vi "Insts_post.vi"(2 "Initialize sweep instruments ??":u64[](array[numeric]), 4 "Initialize readout instruments??":u64[](array[numeric]), 5 "Inst_array":T1(array[cluster])) -> ()   [LabVIEW 2013]
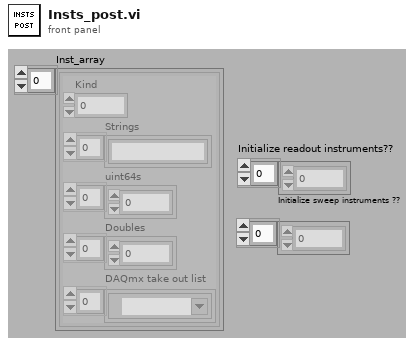
[diagram p1: front panel]
types:
  T1 = cluster{"Kind":u16, "Strings":string[], "uint64s":u64[], "Doubles":dbl[], "DAQmx take out list":refnum<k21>[]}[]
  T2 = cluster{"Kind":u16, "Strings":string[], "uint64s":u64[], "Doubles":dbl[], "DAQmx take out list":refnum<k21>[]}
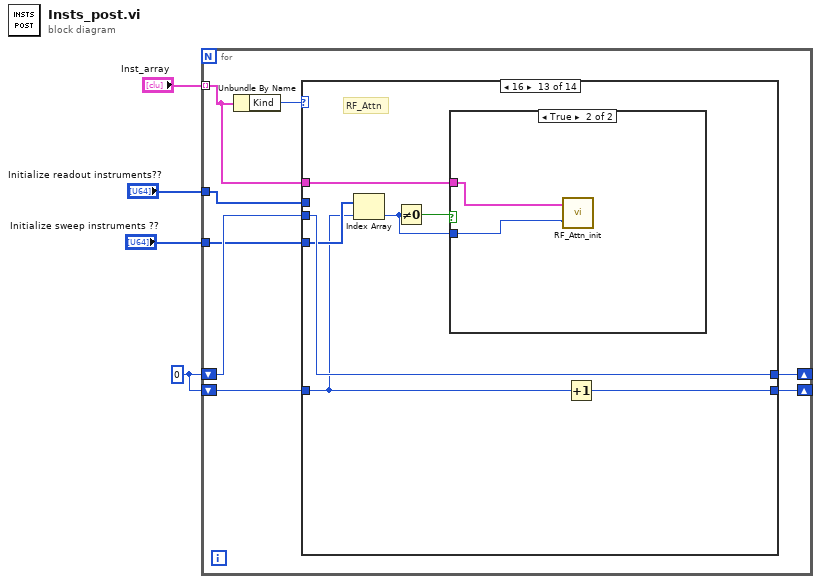
[diagram p0: block diagram]
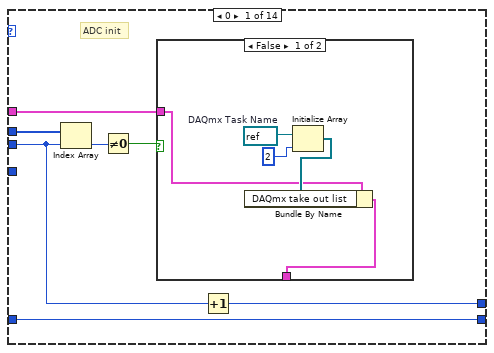
[diagram p2: hidden frame]
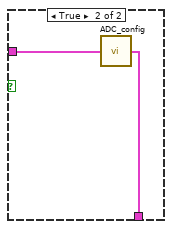
[diagram p3: hidden frame]
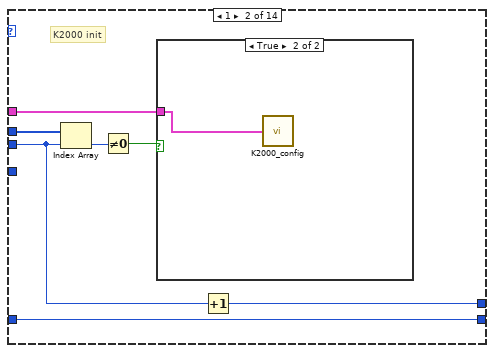
[diagram p4: hidden frame]
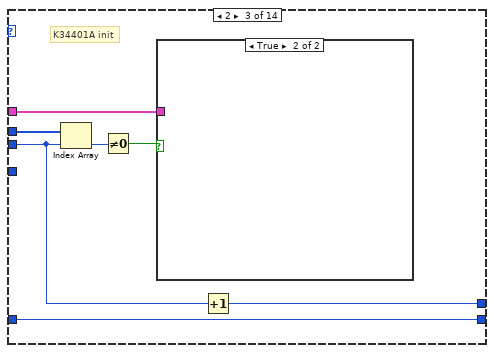
[diagram p6: hidden frame]
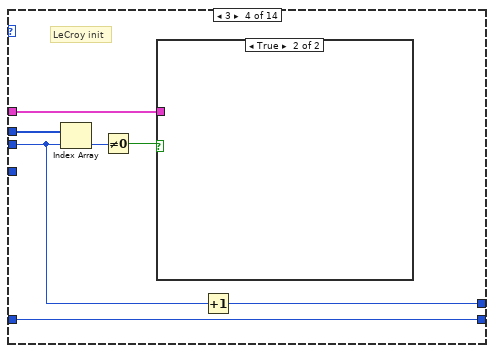
[diagram p8: hidden frame]
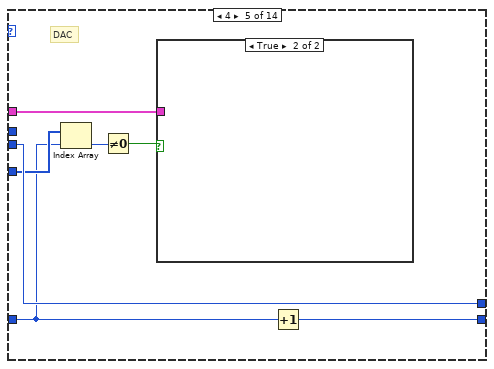
[diagram p10: hidden frame]
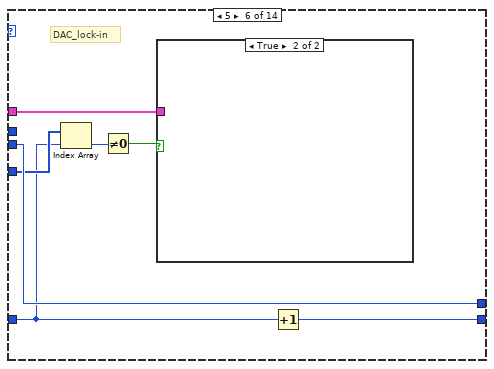
[diagram p12: hidden frame]
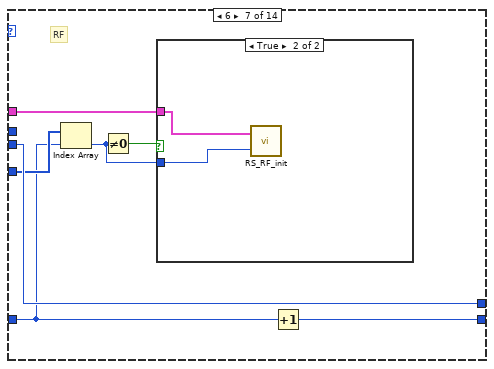
[diagram p14: hidden frame]
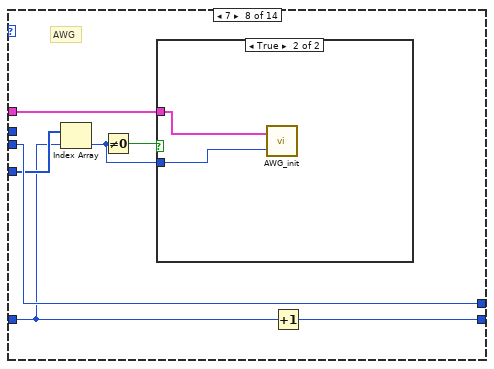
[diagram p16: hidden frame]
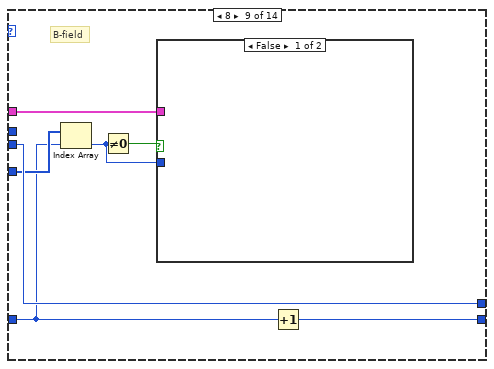
[diagram p18: hidden frame]
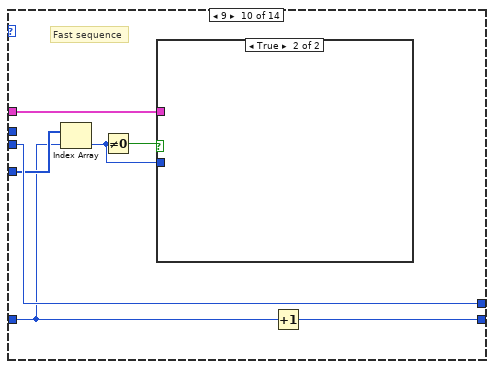
[diagram p20: hidden frame]
diagram:
  w1 = 0
  n1 = for {
    tunnel: "Inst_array" -> [w9] mode=indexing
    tunnel: "Initialize sweep instruments ??" -> [w6]
    tunnel: "Initialize readout instruments??" -> [w10]
    shift-right: [w8] -> _
    shift-left: w1 -> [w11]
    shift-right: [w5] -> _
    shift-left: w1 -> [w7]
    n2 = Unbundle By Name(w9) -> ("Kind"=w12:u16)
    n3 = case shown="16" w12 {
      tunnel: w11 -> [w15 w30 w38 w45 w53 w60 w68 w77 w86 w93 w100 w107 w114 w119]
      tunnel: w10 -> [w19 w33 w41 w48 _ _ _ _ _ _ _ _ _ _]
      tunnel: w9 -> [w16 w28 w36 w43 w49 w56 w64 w73 w82 w89 w96 w103 w110 _]
      tunnel: [w14 w29 w37 w44 w53 w60 w68 w77 w86 w93 w100 w107 w114 w119] -> w8
      tunnel: w7 -> [w13 w27 w35 w42 w50 w57 w65 w74 w83 w90 w97 w104 w111 w118]
      tunnel: w6 -> [_ _ _ _ w52 w59 w67 w76 w85 w92 w99 w106 w113 _]
      tunnel: [w13 w27 w35 w42 w51 w58 w66 w75 w84 w91 w98 w105 w112 w118] -> w5
      frame 0 {
        # "ADC init"
        n4 = Index Array(array=w19, index=w15) -> (element=w18:u64)
        n5 = Not Equal To 0?(x=w18) -> (x != 0?=w17:bool)
        n6 = case shown="False" w17 {
          tunnel: w16 -> [w21 w26]
          tunnel: [w20 w25] -> _
          frame False {
            w24 = refnum<k21> refnum  # DAQmx Task Name
            n7 = Initialize Array(w24, 2) -> (w22:refnum<k21>[])
            n8 = Bundle By Name(cluster=w21, "DAQmx take out list"=w22) -> (w20:T2)
          }
          frame True {
            n9 = call "ADC_config.vi"("Inst_parameter"=w26) -> ("Inst_parameter out"=w25:T2)
          }
        }
        n10 = Increment(x=w15) -> (x+1=w14:i32)
      }
      frame 1 {
        # "K2000 init"
        n11 = Index Array(array=w33, index=w30) -> (element=w32:u64)
        n12 = Not Equal To 0?(x=w32) -> (x != 0?=w31:bool)
        n13 = case shown="True" w31 {
          tunnel: w28 -> [_ w34]
          frame False {
          }
          frame True {
            n14 = call "K2000_config.vi"("Readout_inst_parameters"=w34) -> ()  [unwired: 1 out]
          }
        }
        n15 = Increment(x=w30) -> (x+1=w29:i32)
      }
      frame 2 {
        # "K34401A init"
        n16 = Index Array(array=w41, index=w38) -> (element=w40:u64)
        n17 = Not Equal To 0?(x=w40) -> (x != 0?=w39:bool)
        n18 = case shown="True" w39 {
          tunnel: w36 -> [_ _]
          frame False {
          }
          frame True {
          }
        }
        n19 = Increment(x=w38) -> (x+1=w37:i32)
      }
      frame 3 {
        # "LeCroy init"
        n20 = Index Array(array=w48, index=w45) -> (element=w47:u64)
        n21 = Not Equal To 0?(x=w47) -> (x != 0?=w46:bool)
        n22 = case shown="True" w46 {
          tunnel: w43 -> [_ _]
          frame False {
          }
          frame True {
          }
        }
        n23 = Increment(x=w45) -> (x+1=w44:i32)
      }
      frame 4 {
        # "DAC"
        n24 = Index Array(array=w52, index=w50) -> (element=w55:u64)
        n25 = Not Equal To 0?(x=w55) -> (x != 0?=w54:bool)
        n26 = case shown="True" w54 {
          tunnel: w49 -> [_ _]
          frame False {
          }
          frame True {
          }
        }
        n27 = Increment(x=w50) -> (x+1=w51:i32)
      }
      frame 5 {
        # "DAC_lock-in"
        n28 = Index Array(array=w59, index=w57) -> (element=w62:u64)
        n29 = Not Equal To 0?(x=w62) -> (x != 0?=w61:bool)
        n30 = case shown="True" w61 {
          tunnel: w56 -> [_ _]
          frame False {
          }
          frame True {
          }
        }
        n31 = Increment(x=w57) -> (x+1=w58:i32)
      }
      frame 6 {
        # "RF"
        n32 = Index Array(array=w67, index=w65) -> (element=w63:u64)
        n33 = Not Equal To 0?(x=w63) -> (x != 0?=w69:bool)
        n34 = case shown="True" w69 {
          tunnel: w64 -> [_ w71]
          tunnel: w63 -> [_ w70]
          frame False {
          }
          frame True {
            n35 = call "RS_RF_init.vi"("Initialize Instrument"=w70, "Inst_param"=w71) -> ()  [unwired: 1 in]
          }
        }
        n36 = Increment(x=w65) -> (x+1=w66:i32)
      }
      frame 7 {
        # "AWG"
        n37 = Index Array(array=w76, index=w74) -> (element=w72:u64)
        n38 = Not Equal To 0?(x=w72) -> (x != 0?=w78:bool)
        n39 = case shown="True" w78 {
          tunnel: w73 -> [_ w80]
          tunnel: w72 -> [_ w79]
          frame False {
          }
          frame True {
            n40 = call "AWG_init.vi"("Initialize?"=w79, "Inst_param"=w80) -> ()  [unwired: 1 out]
          }
        }
        n41 = Increment(x=w74) -> (x+1=w75:i32)
      }
      frame 8 {
        # "B-field"
        n42 = Index Array(array=w85, index=w83) -> (element=w81:u64)
        n43 = Not Equal To 0?(x=w81) -> (x != 0?=w87:bool)
        n44 = case shown="False" w87 {
          tunnel: w82 -> [_ _]
          tunnel: w81 -> [_ _]
          frame False {
          }
          frame True {
          }
        }
        n45 = Increment(x=w83) -> (x+1=w84:i32)
      }
      frame 9 {
        # "Fast sequence"
        n46 = Index Array(array=w92, index=w90) -> (element=w88:u64)
        n47 = Not Equal To 0?(x=w88) -> (x != 0?=w94:bool)
        n48 = case shown="True" w94 {
          tunnel: w89 -> [_ _]
          tunnel: w88 -> [_ _]
          frame False {
          }
          frame True {
          }
        }
        n49 = Increment(x=w90) -> (x+1=w91:i32)
      }
      frame 10 {
        # "Fast sequence slot"
        n50 = Index Array(array=w99, index=w97) -> (element=w95:u64)
        n51 = Not Equal To 0?(x=w95) -> (x != 0?=w101:bool)
        n52 = case shown="True" w101 {
          tunnel: w96 -> [_ _]
          tunnel: w95 -> [_ _]
          frame False {
          }
          frame True {
          }
        }
        n53 = Increment(x=w97) -> (x+1=w98:i32)
      }
      frame 11 {
        # "Command line"
        n54 = Index Array(array=w106, index=w104) -> (element=w102:u64)
        n55 = Not Equal To 0?(x=w102) -> (x != 0?=w108:bool)
        n56 = case shown="True" w108 {
          tunnel: w103 -> [_ _]
          tunnel: w102 -> [_ _]
          frame False {
          }
          frame True {
          }
        }
        n57 = Increment(x=w104) -> (x+1=w105:i32)
      }
      frame 16 {
        # "RF_Attn"
        n58 = Index Array(array=w113, index=w111) -> (element=w109:u64)
        n59 = Not Equal To 0?(x=w109) -> (x != 0?=w115:bool)
        n60 = case shown="True" w115 {
          tunnel: w110 -> [_ w117]
          tunnel: w109 -> [_ w116]
          frame False {
          }
          frame True {
            n61 = call "RF_Attn_init.vi"("Initialize Instrument"=w116, "Inst_param"=w117) -> ()  [unwired: 1 in]
          }
        }
        n62 = Increment(x=w111) -> (x+1=w112:i32)
      }
      frame 100, Default {
        # "Else"
      }
    }
  }
